vi "Action Message Loop.vi"(7 "Measurement UI Controls":T1 caption="测量UI控件", 8 "error in (no error)":errorcluster caption="错误输入（无错误）", 10 "Data Notifier":refnum<notifier> caption="数据通知器", 11 "Message Queues":T2 caption="消息队列") -> (0 "error out":errorcluster caption="错误输出")   [LabVIEW 2015, in "Action.lvlib"]
doc: "该消息循环负责处理硬件数据采集的相关消息。"
uses:
  Action.lvlib
  <vilib>/Utility/error.llb/Error Cluster From Error Code.vi
  support/Message Queue/Message Queue.lvlib
  support/Message Queue/Enqueue Message (Single).vi
  <vilib>/ErrorRing/Error Ring.xnode
  Acquisition State.ctl
  Hardware Configuration.ctl
  Measure/Measure Type.ctl
  support/Message Queue/Message Cluster.ctl
  support/Message Queue/All Message Queues.ctl
  controls/UI Data.ctl
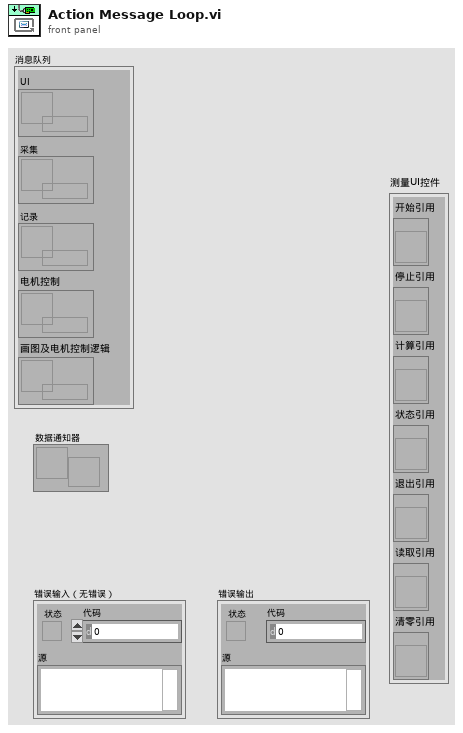
[diagram p1: front panel]
types:
  T1 = typedef "UI Data.ctl" = cluster{"Start Ref":refnum<vi>, "Stop Ref":refnum<vi>, "calculate Ref":refnum<vi>, "Status Ref":refnum<vi>, "Exit Ref":refnum<vi>, "read Ref":refnum<vi>, "clean Ref":refnum<vi>}
  T2 = typedef "Message Queue.lvlib/All Message Queues.ctl" = cluster{"UI":refnum<queue>, "Acquisition":refnum<queue>, "Logging":refnum<queue>, "plot logic":refnum<queue>, "Action Control":refnum<queue>}
  T3 = typedef "Action.lvlib/Hardware Configuration.ctl" = cluster{"PLC设置":T4, "动作设置":T5, "电机设置":T9, "所有测试电机转动逻辑":T10}
  T4 = typedef "Action.lvlib/PLC设置.ctl" = cluster{"ActLogicalStationNumber":i32, "ActUtlType":refnum<k7>}
  T5 = typedef "Action.lvlib/动作设置.ctl" = cluster{"自动跳法测试动作":T6, "其他动作":T8}
  T6 = typedef "Action.lvlib/自动调阀测试动作设置.ctl" = cluster{"夹紧/松阀总":T7, "夹紧/松阀齿":T7, "方向机供油":T7, "扭杆紧/松":T7, "压销":cluster{"PLC指令":T7}}
  T7 = typedef "Action.lvlib/PLC控制指令.ctl" = cluster{"变量类型":u32, "PLC地址":i32, "size":i32, "写入数据(写入时有效)":i16}
  T8 = typedef "Action.lvlib/其他动作设置 .ctl" = cluster{"其他指令1":T7, "其他指令2":T7, "其他指令3":T7, "其他指令4":T7, "其他指令5":T7}
  T9 = typedef "Action.lvlib/电机控制设置.ctl" = cluster{"counter":tag, "方向端口":tag, "当前方向":bool, "频率":dbl, "DAQmx Task":refnum<k21>}
  T10 = typedef "Action.lvlib/所有测试电机转动逻辑.ctl" = cluster{"啮合测试电机转动逻辑":T11, "退回测试电机转动逻辑":T11, "功能测试电机转动逻辑":T11, "力特性测试电机转动逻辑":T11, "自动调阀测试分中电机转动逻辑":T11, "自动调阀测试对中电机转动逻辑":T11}
  T11 = typedef "Action.lvlib/电机转动逻辑1.ctl" = cluster{"反转判断条件1":T12, "停止判断条件1":T13}
  T12 = typedef "Action.lvlib/反转判断条件1.ctl" = cluster{"传感器序号":i32, "条件":enum16{"小于", "大于", "等于"}, "值":dbl, "条件判断时间间隔":i32, "反转等待时长":i32}
  T13 = typedef "Action.lvlib/停止判断条件1.ctl" = cluster{"角度传感器序号":i32, "正转/反转":enum16{"正转", "反转"}, "反转次数":i32, "停止角度":dbl, "停止角度误差范围":dbl}
  T14 = typedef "Measure Type.ctl" = enum16{"啮合", "退回", "功能", "力特性", "内泄漏", "自动调阀测试"}
  T15 = typedef "Action.lvlib/Acquisition State.ctl" = enum16{"Idle", "Acquiring"}
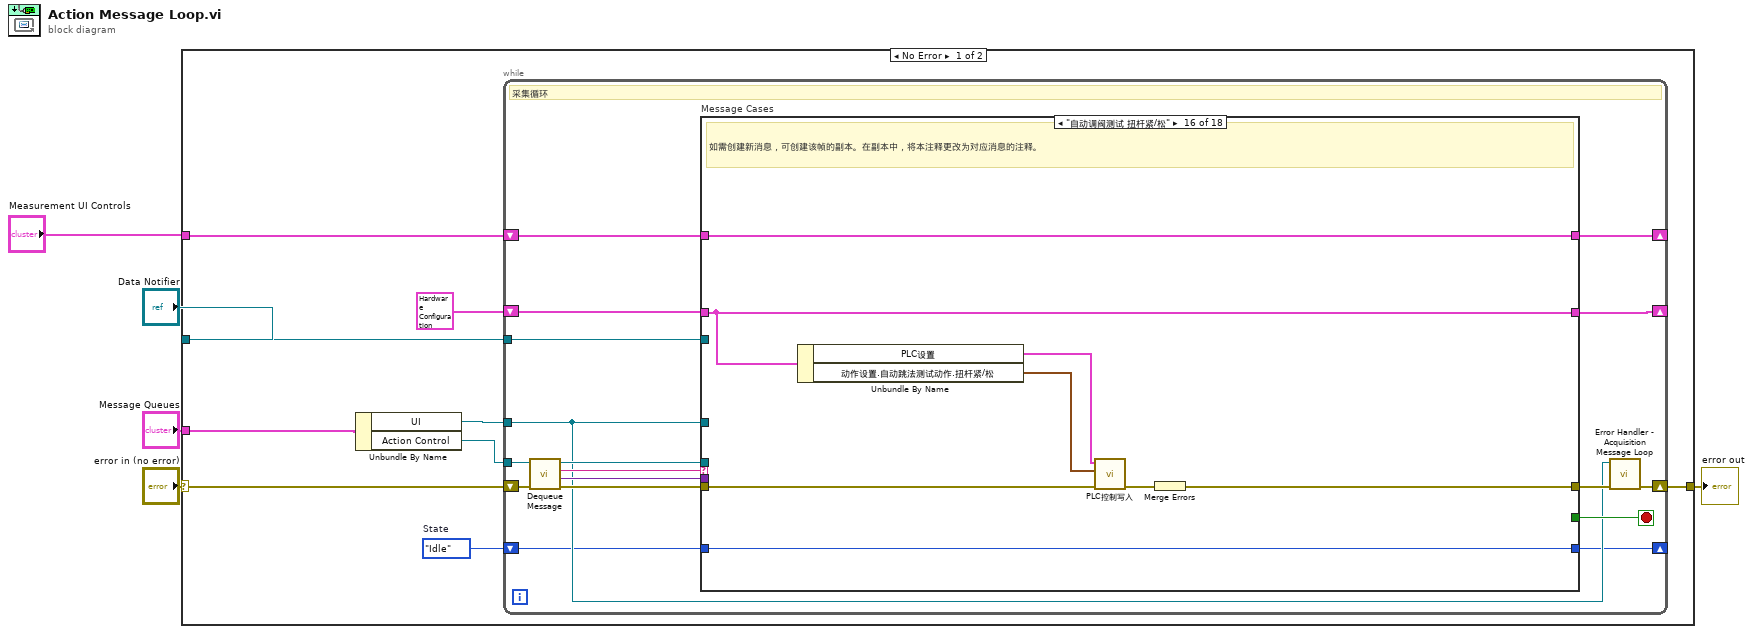
[diagram p0: block diagram]
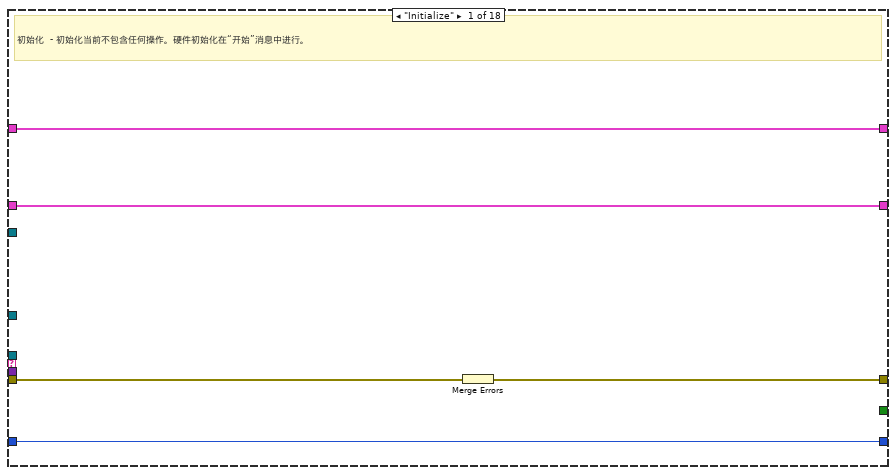
[diagram p2: hidden frame]
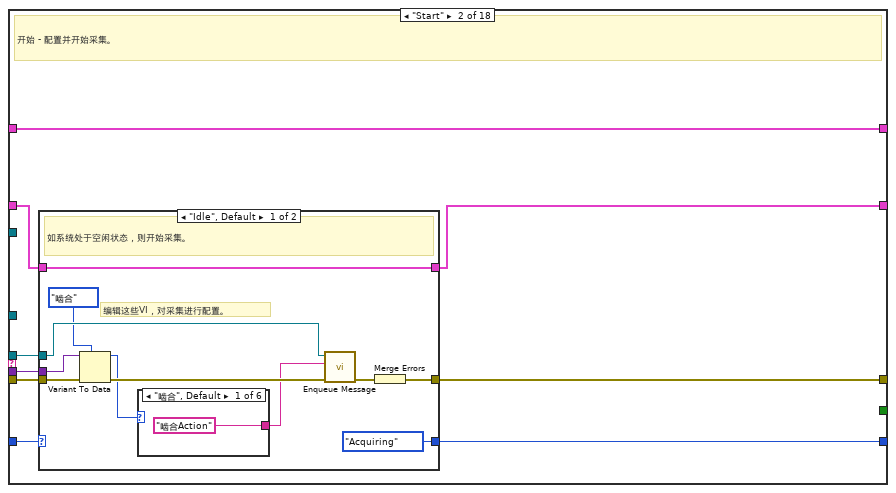
[diagram p3: hidden frame]
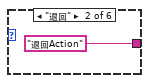
[diagram p4: hidden frame]
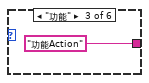
[diagram p5: hidden frame]
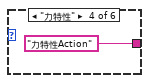
[diagram p6: hidden frame]
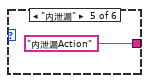
[diagram p7: hidden frame]
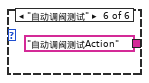
[diagram p8: hidden frame]
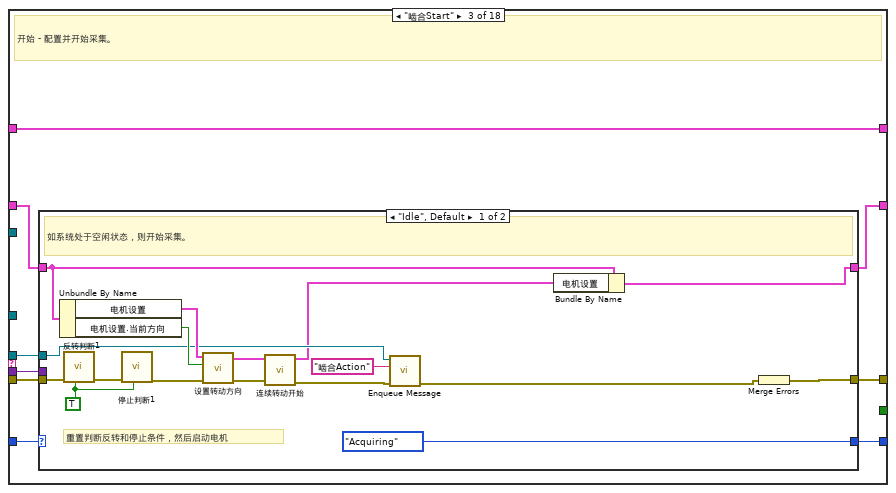
[diagram p10: hidden frame]
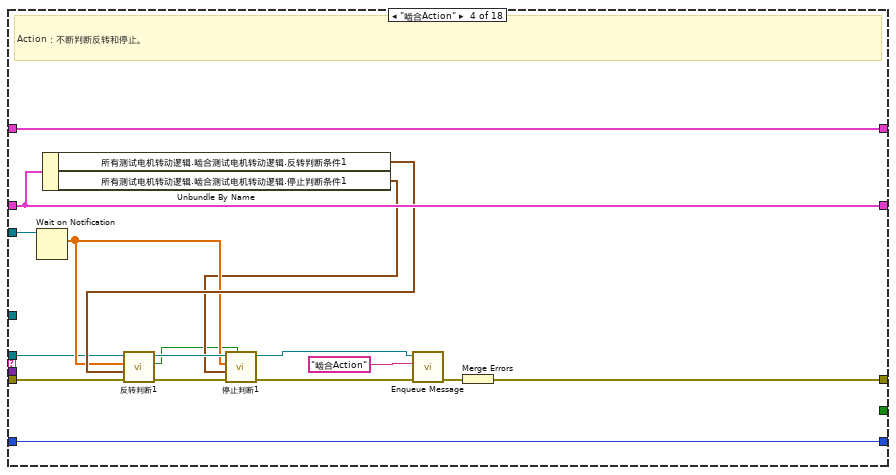
[diagram p12: hidden frame]
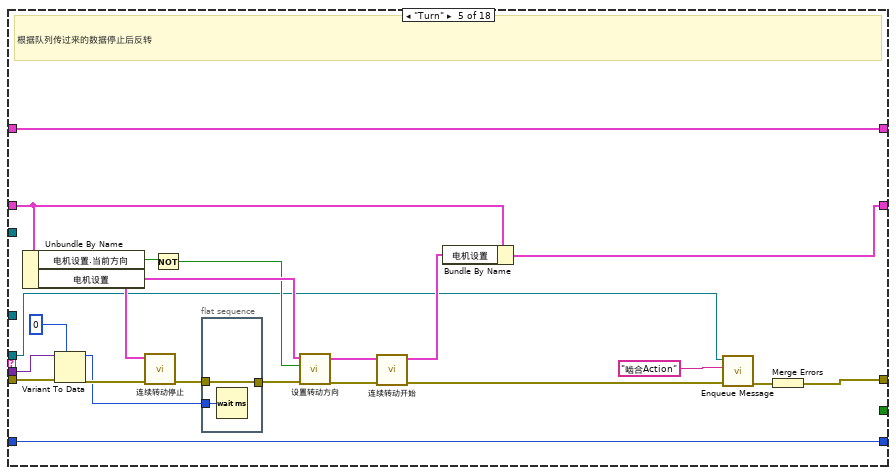
[diagram p13: hidden frame]
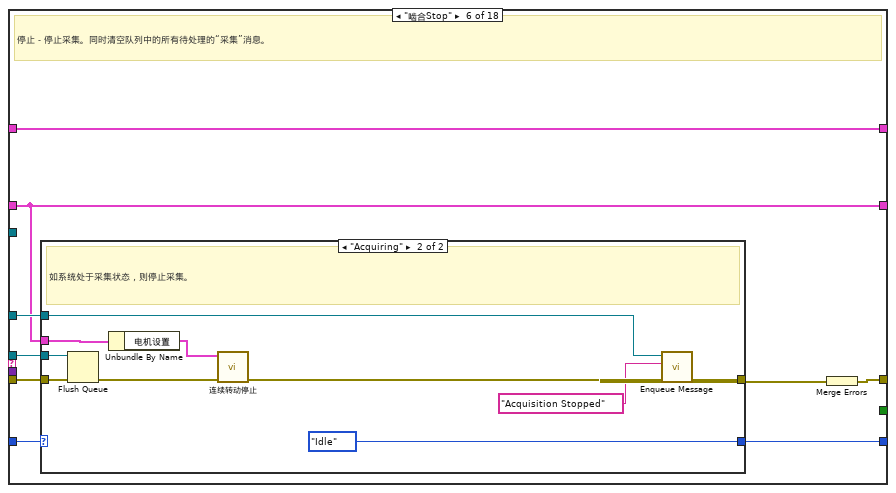
[diagram p14: hidden frame]
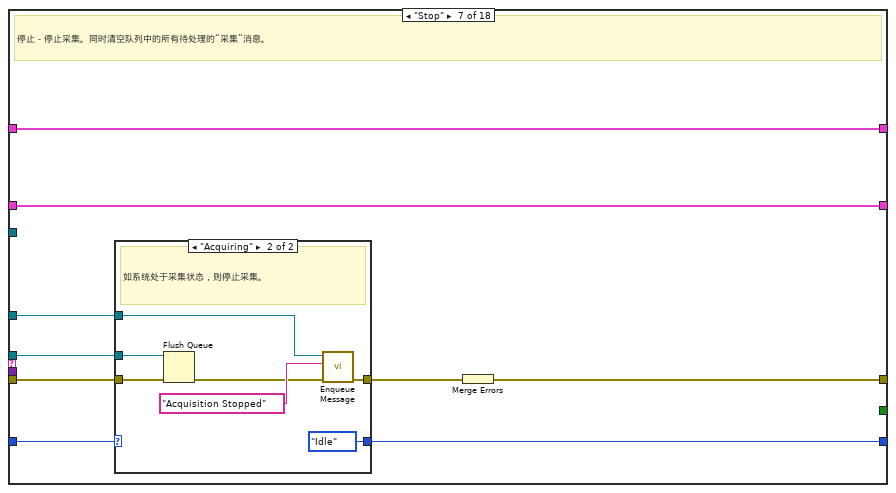
[diagram p16: hidden frame]
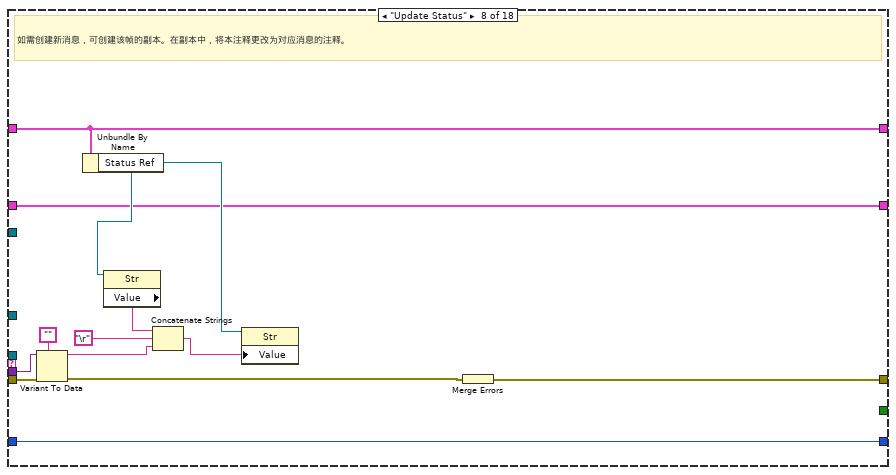
[diagram p18: hidden frame]
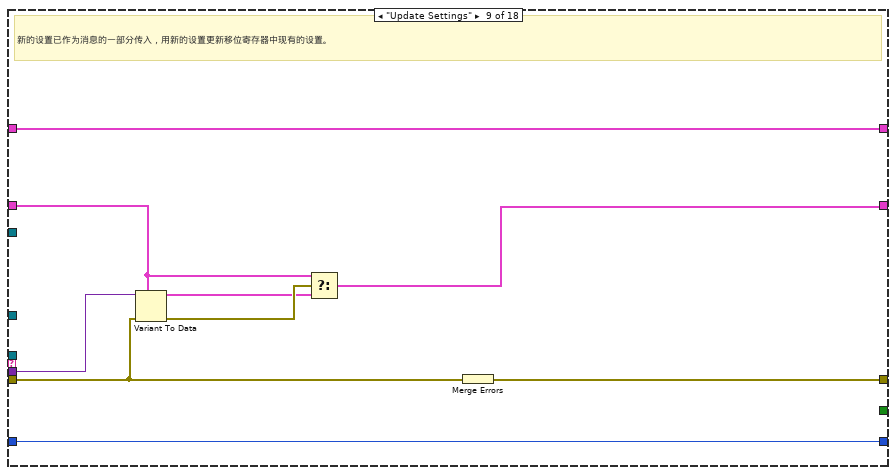
[diagram p19: hidden frame]
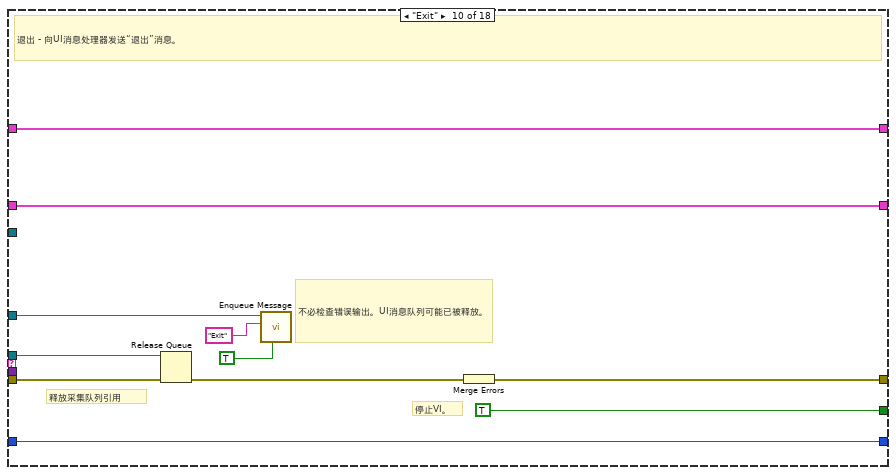
[diagram p20: hidden frame]
diagram:
  n1 = case shown="No Error" "error in (no error)" {
    selector: "error in (no error)" -> [w11 w294]
    tunnel: "Message Queues" -> [w14 _]
    tunnel: [w12 w294] -> w4
    tunnel: "Data Notifier" -> [w9 _]
    tunnel: "Measurement UI Controls" -> [w7 _]
    frame No Error {
      w8 = Acquisition_State."Idle"  # State
      n2 = Unbundle By Name(w14) -> ("UI"=w10:refnum<queue>, "Action Control"=w13:refnum<queue>)
      n3 = while {
        tunnel: w13 -> [w25]
        shift-right: [w22] -> w12
        shift-left: w11 -> [w30]
        tunnel: w10 -> [w21]
        tunnel: w9 -> [w24]
        shift-right: [w19] -> _
        shift-left: w8 -> [w20]
        shift-right: [w15] -> _
        shift-left: w7 -> [w18]
        shift-right: [w16] -> _
        shift-left: T3 {"PLC设置"={"ActLogicalStationNumber"=9600, "ActUtlType"=refnum}, "动作设置"={"自动跳法测试动作"={"夹紧/松阀总"={"变量类型"=2, "PLC地址"=0, "size"=0, "写入数据(写入时有效)"=0}, "夹紧/松阀齿"={"变量类型"=2, "PLC地址"=0, "size"=0, "写入数据(写入时有效)"=0}, "方向机供油"={"变量类型"=2, "PLC地址"=0, "size"=0, "写入数据(写入时有效)"=0}, "扭杆紧/松"={"变量类型"=2, "PLC地址"=0, "size"=0, "写入数据(写入时有效)"=0}, "压销"={"PLC指令"={"变量类型"=2, "PLC地址"=0, "size"=0, "写入数据(写入时有效)"=0}}}, "其他动作"={"其他指令1"={"变量类型"=2, "PLC地址"=0, "size"=0, "写入数据(写入时有效)"=0}, "其他指令2"={"变量类型"=2, "PLC地址"=0, "size"=0, "写入数据(写入时有效)"=0}, "其他指令3"={"变量类型"=2, "PLC地址"=0, "size"=0, "写入数据(写入时有效)"=0}, "其他指令4"={"变量类型"=2, "PLC地址"=0, "size"=0, "写入数据(写入时有效)"=0}, "其他指令5"={"变量类型"=2, "PLC地址"=0, "size"=0, "写入数据(写入时有效)"=0}}}, "电机设置"={"counter"="Dev1/ctr0", "方向端口"="", "当前方向"=FALSE, "频率"=0.0, "DAQmx Task"=""}, "所有测试电机转动逻辑"={"啮合测试电机转动逻辑"={"反转判断条件1"={"传感器序号"=0, "条件"=enum."小于", "值"=0.0, "条件判断时间间隔"=0, "反转等待时长"=0}, "停止判断条件1"={"角度传感器序号"=0, "正转/反转"=enum."正转", "反转次数"=0, "停止角度"=0.0, "停止角度误差范围"=0.0}}, "退回测试电机转动逻辑"={"反转判断条件1"={"传感器序号"=0, "条件"=enum."小于", "值"=0.0, "条件判断时间间隔"=0, "反转等待时长"=0}, "停止判断条件1"={"角度传感器序号"=0, "正转/反转"=enum."正转", "反转次数"=0, "停止角度"=0.0, "停止角度误差范围"=0.0}}, "功能测试电机转动逻辑"={"反转判断条件1"={"传感器序号"=0, "条件"=enum."小于", "值"=0.0, "条件判断时间间隔"=0, "反转等待时长"=0}, "停止判断条件1"={"角度传感器序号"=0, "正转/反转"=enum."正转", "反转次数"=0, "停止角度"=0.0, "停止角度误差范围"=0.0}}, "力特性测试电机转动逻辑"={"反转判断条件1"={"传感器序号"=0, "条件"=enum."小于", "值"=0.0, "条件判断时间间隔"=0, "反转等待时长"=0}, "停止判断条件1"={"角度传感器序号"=0, "正转/反转"=enum."正转", "反转次数"=0, "停止角度"=0.0, "停止角度误差范围"=0.0}}, "自动调阀测试分中电机转动逻辑"={"反转判断条件1"={"传感器序号"=0, "条件"=enum."小于", "值"=0.0, "条件判断时间间隔"=0, "反转等待时长"=0}, "停止判断条件1"={"角度传感器序号"=0, "正转/反转"=enum."正转", "反转次数"=0, "停止角度"=0.0, "停止角度误差范围"=0.0}}, "自动调阀测试对中电机转动逻辑"={"反转判断条件1"={"传感器序号"=0, "条件"=enum."小于", "值"=0.0, "条件判断时间间隔"=0, "反转等待时长"=0}, "停止判断条件1"={"角度传感器序号"=0, "正转/反转"=enum."正转", "反转次数"=0, "停止角度"=0.0, "停止角度误差范围"=0.0}}}} ("Hardware Configuration") -> [w17]
        stop <- w31 stop-if-true
        # "采集循环"
        n4 = call "Dequeue Message.vi"("error in (no error)"=w30, "Message Queue"=w25) -> ("error out"=w29:errorcluster, "Message Data"=w27:variant, "Message"=w28:string, "dup Message Queue"=w26:refnum<queue>)  [unwired: 6 in]
        n5 = case "Message Cases" shown="\"自动调阀测试 扭杆紧/松\"" w28 {
          selector: w28 -> [_ _ _ _ _ _ _ _ _ _ w212 _ _ _ _ _ _ _]
          tunnel: w26 -> [_ w42 w71 w97 w112 w142 w163 _ _ w200 _ _ _ _ _ _ w262 _]
          tunnel: w29 -> [w35 w43 w72 w103 w128 w143 w164 w184 w194 w204 _ w224 w230 w238 w246 w254 w263 w291]
          tunnel: [w36 w45 w74 w111 w133 w144 w165 w187 w196 w206 w211 w223 w232 w240 w248 w256 w265 w293] -> w23
          tunnel: w17 -> [w33 w44 w73 w106 w115 w136 w158 w176 w190 w198 w209 w221 w226 w234 w242 w250 w264 w287]
          tunnel: [_ _ _ _ _ _ _ _ _ TRUE _ _ _ _ _ _ _ _] -> w31
          tunnel: w27 -> [_ w37 w66 _ w127 _ _ w183 w192 _ _ _ _ _ _ _ w257 _]
          tunnel: w21 -> [_ _ _ _ _ w141 w162 _ _ w205 _ _ _ _ _ _ _ _]
          tunnel: w24 -> [_ _ _ w104 _ _ _ _ _ _ _ _ _ _ _ _ _ _]
          tunnel: w20 -> [w34 w41 w70 w108 w130 w140 w161 w186 w193 w199 w210 w222 w231 w239 w247 w255 w261 w292]
          tunnel: [w34 w40 w69 w108 w130 w139 w160 w186 w193 w199 w210 w222 w231 w239 w247 w255 w260 w292] -> w19
          tunnel: w18 -> [w32 w38 w67 w107 w129 w137 w157 w175 w188 w197 w208 w220 w225 w233 w241 w249 w258 w286]
          tunnel: [w33 w39 w68 w106 w113 w136 w158 w176 w189 w198 w209 w221 w226 w234 w242 w250 w259 w287] -> w16
          tunnel: [w32 w38 w67 w107 w129 w137 w157 w175 w188 w197 w208 w220 w225 w233 w241 w249 w258 w286] -> w15
          frame "Initialize" {
            # "初始化  - 初始化当前不包含任何操作。硬件初始化在“开始”消息中进行。"
            n6 = Merge Errors(w35) -> (w36:errorcluster)
          }
          frame "Start" {
            # "开始 - 配置并开始采集。"
            n7 = case shown="\"Idle\", Default" w41 {
              selector: w41 -> [_ w63]
              tunnel: [w56 w65] -> w45
              tunnel: w44 -> [w52 w64]
              tunnel: w43 -> [w51 w65]
              tunnel: w42 -> [w54 _]
              tunnel: [w52 w64] -> w39
              tunnel: [Acquisition_State."Acquiring" ("State") w63] -> w40
              tunnel: w37 -> [w49 _]
              frame "Idle", Default {
                # "编辑这些VI，对采集进行配置。"
                # "如系统处于空闲状态，则开始采集。"
                n8 = Variant To Data(error in=w51, type=Measure_Type."啮合" ("测试类型"), Variant=w49) -> (data=w47:T14, error out=w50:errorcluster)
                n9 = case shown="\"啮合\", Default" w47 {
                  tunnel: ["啮合Action" ("Message") "退回Action" ("Message") "功能Action" ("Message") "力特性Action" ("Message") "内泄漏Action" ("Message") "自动调阀测试Action" ("Message")] -> w46
                  frame "啮合", Default {
                  }
                  frame "退回" {
                  }
                  frame "功能" {
                  }
                  frame "力特性" {
                  }
                  frame "内泄漏" {
                  }
                  frame "自动调阀测试" {
                  }
                }
                n10 = call-poly "Enqueue Message.vi"("error in (no error)"=w50, "Message"=w46, "Message Queue"=w54) -> ("error out"=w55:errorcluster)  [unwired: 7 in, 1 out]
                n11 = Merge Errors(w55) -> (w56:errorcluster)
              }
              frame "Acquiring" {
                # "系统已开始采集。忽略“开始”消息。"
              }
            }
          }
          frame "啮合Start" {
            # "开始 - 配置并开始采集。"
            n12 = case shown="\"Idle\", Default" w70 {
              selector: w70 -> [_ w92]
              tunnel: [w91 w94] -> w74
              tunnel: w73 -> [w77 w93]
              tunnel: w72 -> [w86 w94]
              tunnel: w71 -> [w79 _]
              tunnel: [w75 w93] -> w68
              tunnel: [Acquisition_State."Acquiring" ("State") w92] -> w69
              tunnel: w66 -> [_ _]
              frame "Idle", Default {
                w87 = TRUE ("重置？")
                # "重置判断反转和停止条件，然后启动电机"
                # "如系统处于空闲状态，则开始采集。"
                n13 = Unbundle By Name(w77) -> ("电机设置"=w83:T9, "电机设置.当前方向"=w84:bool)
                n14 = call "反转判断1.vi"("重置？"=w87, "error in (no error)"=w86) -> ("error out"=w88:errorcluster)  [unwired: 7 in, 2 out]
                n15 = call "停止判断1.vi"("重置？"=w87, "error in (no error)"=w88) -> ("error out"=w85:errorcluster)  [unwired: 8 in, 1 out]
                n16 = call "设置转动方向.vi"("error in (no error)"=w85, "方向"=w84, "Hardware Resources in"=w83) -> ("error out"=w82:errorcluster, "Hardware Resources out"=w81:T9)  [unwired: 7 in]
                n17 = call "连续转动开始.vi"("error in (no error)"=w82, "Hardware Resources in"=w81) -> ("error out"=w80:errorcluster, "Hardware Resources out"=w76:T9)  [unwired: 8 in]
                n18 = call-poly "Enqueue Message.vi"("error in (no error)"=w80, "Message"="啮合Action", "Message Queue"=w79) -> ("error out"=w78:errorcluster)  [unwired: 7 in, 1 out]
                n19 = Bundle By Name(cluster=w77, "电机设置"=w76) -> (w75:T3)
                n20 = Merge Errors(w78) -> (w91:errorcluster)
              }
              frame "Acquiring" {
                # "系统已开始采集。忽略“开始”消息。"
              }
            }
          }
          frame "啮合Action" {
            # "Action：不断判断反转和停止。"
            n21 = Wait on Notification(notifier=w104) -> (notification=w100:dbl[])  [unwired: 3 in, 3 out]
            n22 = Unbundle By Name(w106) -> ("所有测试电机转动逻辑.啮合测试电机转动逻辑.反转判断条件1"=w105:T12, "所有测试电机转动逻辑.啮合测试电机转动逻辑.停止判断条件1"=w99:T13)
            n23 = call "反转判断1.vi"("error in (no error)"=w103, "反转判断条件1"=w105, "传感器数据"=w100, "Message Queue"=w97) -> ("error out"=w102:errorcluster, "反转"=w98:bool, "Message Queue 2"=w101:refnum<queue>)  [unwired: 5 in]
            n24 = call "停止判断1.vi"("反转？"=w98, "error in (no error)"=w102, "反转判断条件1"=w99, "传感器数据"=w100, "Message Queue"=w101) -> ("error out"=w95:errorcluster, "Message Queue 2"=w96:refnum<queue>)  [unwired: 5 in]
            n25 = call-poly "Enqueue Message.vi"("error in (no error)"=w95, "Message"="啮合Action", "Message Queue"=w96) -> ("error out"=w110:errorcluster)  [unwired: 7 in, 1 out]
            n26 = Merge Errors(w110) -> (w111:errorcluster)
          }
          frame "Turn" {
            # "根据队列传过来的数据停止后反转"
            n27 = Unbundle By Name(w115) -> ("电机设置.当前方向"=w120:bool, "电机设置"=w121:T9)
            n28 = Variant To Data(error in=w128, type=0, Variant=w127) -> (data=w124:i32, error out=w125:errorcluster)
            n29 = call "连续转动停止.vi"("error in (no error)"=w125, "Hardware Resources in"=w121) -> ("error out"=w123:errorcluster)  [unwired: 9 in]
            n30 = Not(x=w120) -> (.not. x?=w119:bool)
            n31 = flat-sequence {
              tunnel: w124 -> [w135]
              tunnel: [w134] -> w122
              tunnel: w123 -> [w134]
              frame #0 {
                n32 = Wait (ms)(milliseconds to wait=w135) -> ()  [unwired: 1 out]
              }
            }
            n33 = call "设置转动方向.vi"("error in (no error)"=w122, "方向"=w119, "Hardware Resources in"=w121) -> ("error out"=w118:errorcluster, "Hardware Resources out"=w117:T9)  [unwired: 7 in]
            n34 = call "连续转动开始.vi"("error in (no error)"=w118, "Hardware Resources in"=w117) -> ("error out"=w116:errorcluster, "Hardware Resources out"=w114:T9)  [unwired: 8 in]
            n35 = Bundle By Name(cluster=w115, "电机设置"=w114) -> (w113:T3)
            n36 = call-poly "Enqueue Message.vi"("error in (no error)"=w116, "Message"="啮合Action", "Message Queue"=w112) -> ("error out"=w132:errorcluster)  [unwired: 7 in, 1 out]
            n37 = Merge Errors(w132) -> (w133:errorcluster)
          }
          frame "啮合Stop" {
            # "停止－停止采集。同时清空队列中的所有待处理的“采集”消息。"
            n38 = case shown="\"Acquiring\"" w140 {
              selector: w140 -> [w146 _]
              tunnel: w143 -> [w145 w156]
              tunnel: w142 -> [_ w155]
              tunnel: w141 -> [_ w154]
              tunnel: [w146 Acquisition_State."Idle" ("State")] -> w139
              tunnel: [w145 w153] -> w138
              tunnel: w136 -> [_ w149]
              frame "Idle", Default {
                # "系统已处于空闲状态。忽略“停止”消息。"
              }
              frame "Acquiring" {
                # "如系统处于采集状态，则停止采集。"
                n39 = Flush Queue(queue=w155, error in (no error)=w156) -> (error out=w150:errorcluster)  [unwired: 2 out]
                n40 = Unbundle By Name(w149) -> ("电机设置"=w148:T9)
                n41 = call "连续转动停止.vi"("error in (no error)"=w150, "Hardware Resources in"=w148) -> ("error out"=w147:errorcluster)  [unwired: 9 in]
                n42 = call-poly "Enqueue Message.vi"("error in (no error)"=w147, "Message"="Acquisition Stopped", "Message Queue"=w154) -> ("error out"=w153:errorcluster)  [unwired: 7 in, 1 out]
              }
            }
            n43 = Merge Errors(w138) -> (w144:errorcluster)
          }
          frame "Stop" {
            # "停止－停止采集。同时清空队列中的所有待处理的“采集”消息。"
            n44 = case shown="\"Acquiring\"" w161 {
              selector: w161 -> [w167 _]
              tunnel: w164 -> [w166 w174]
              tunnel: w163 -> [_ w173]
              tunnel: w162 -> [_ w172]
              tunnel: [w167 Acquisition_State."Idle" ("State")] -> w160
              tunnel: [w166 w171] -> w159
              frame "Idle", Default {
                # "系统已处于空闲状态。忽略“停止”消息。"
              }
              frame "Acquiring" {
                # "如系统处于采集状态，则停止采集。"
                n45 = Flush Queue(queue=w173, error in (no error)=w174) -> (error out=w168:errorcluster)  [unwired: 2 out]
                n46 = call-poly "Enqueue Message.vi"("error in (no error)"=w168, "Message"="Acquisition Stopped", "Message Queue"=w172) -> ("error out"=w171:errorcluster)  [unwired: 7 in, 1 out]
              }
            }
            n47 = Merge Errors(w159) -> (w165:errorcluster)
          }
          frame "Update Status" {
            # "如需创建新消息，可创建该帧的副本。在副本中，将本注释更改为对应消息的注释。"
            n48 = Variant To Data(error in=w184, type="", Variant=w183) -> (data=w178:string, error out=w182:errorcluster)
            n49 = Unbundle By Name(w175) -> ("Status Ref"=w181:refnum<vi>)
            n50 = property class="Str"(reference=w181) -> ("Value"=w180:string)  [unwired: 1 in, 2 out]
            n51 = Concatenate Strings(w180, "\r", w178) -> (w177:string)
            n52 = property class="Str"(reference=w181, "Value"=w177) -> ()  [unwired: 1 in, 2 out]
            n53 = Merge Errors(w182) -> (w187:errorcluster)
          }
          frame "Update Settings" {
            # "新的设置已作为消息的一部分传入，用新的设置更新移位寄存器中现有的设置。"
            n54 = Variant To Data(error in=w194, type=w190, Variant=w192) -> (data=w191:T3, error out=w195:errorcluster)
            n55 = Select(t=w190, s=w195, f=w191) -> (s? t:f=w189:T3)
            n56 = Merge Errors(w194) -> (w196:errorcluster)
          }
          frame "Exit" {
            # "不必检查错误输出。UI消息队列可能已被释放。"
            # "释放采集队列引用"
            # "停止VI。"
            # "退出 - 向UI消息处理器发送“退出”消息。"
            n57 = Release Queue(queue=w200, error in (no error)=w204) -> (error out=w201:errorcluster)  [unwired: 1 in, 2 out]
            n58 = call-poly "Enqueue Message.vi"("Priority Message? (F)"=TRUE, "Message"="Exit", "Message Queue"=w205) -> ()  [unwired: 7 in, 2 out]
            n59 = Merge Errors(w201) -> (w206:errorcluster)
          }
          frame Default {
            # "如得到的消息未经任何分支定义，则运行“默认”分支。输出程序错误。"
            n60 = xnode "Error Ring"("parameter 0"=w212) -> ("error out"=w211:errorcluster)
          }
          frame "---Copy This Frame---" {
            # "如需创建新消息，可创建该帧的副本。在副本中，将本注释更改为对应消息的注释。"
            n61 = Merge Errors(w224) -> (w223:errorcluster)
          }
          frame "自动调阀测试 夹紧/松阀总" {
            # "如需创建新消息，可创建该帧的副本。在副本中，将本注释更改为对应消息的注释。"
            n62 = Unbundle By Name(w226) -> ("PLC设置"=w228:T4, "动作设置.自动跳法测试动作.夹紧/松阀总"=w227:T7)
            n63 = call "PLC控制写入.vi"("error in (no error)"=w230, "PLC指令"=w227, "PLC设置"=w228) -> ("error out"=w229:errorcluster)  [unwired: 6 in, 2 out]
            n64 = Merge Errors(w229) -> (w232:errorcluster)
          }
          frame "自动调阀测试 夹紧/松阀齿" {
            # "如需创建新消息，可创建该帧的副本。在副本中，将本注释更改为对应消息的注释。"
            n65 = Unbundle By Name(w234) -> ("PLC设置"=w236:T4, "动作设置.自动跳法测试动作.夹紧/松阀齿"=w235:T7)
            n66 = call "PLC控制写入.vi"("error in (no error)"=w238, "PLC指令"=w235, "PLC设置"=w236) -> ("error out"=w237:errorcluster)  [unwired: 6 in, 2 out]
            n67 = Merge Errors(w237) -> (w240:errorcluster)
          }
          frame "自动调阀测试 方向机供油" {
            # "如需创建新消息，可创建该帧的副本。在副本中，将本注释更改为对应消息的注释。"
            n68 = Unbundle By Name(w242) -> ("PLC设置"=w244:T4, "动作设置.自动跳法测试动作.方向机供油"=w243:T7)
            n69 = call "PLC控制写入.vi"("error in (no error)"=w246, "PLC指令"=w243, "PLC设置"=w244) -> ("error out"=w245:errorcluster)  [unwired: 6 in, 2 out]
            n70 = Merge Errors(w245) -> (w248:errorcluster)
          }
          frame "自动调阀测试 扭杆紧/松" {
            # "如需创建新消息，可创建该帧的副本。在副本中，将本注释更改为对应消息的注释。"
            n71 = Unbundle By Name(w250) -> ("PLC设置"=w252:T4, "动作设置.自动跳法测试动作.扭杆紧/松"=w251:T7)
            n72 = call "PLC控制写入.vi"("error in (no error)"=w254, "PLC指令"=w251, "PLC设置"=w252) -> ("error out"=w253:errorcluster)  [unwired: 6 in, 2 out]
            n73 = Merge Errors(w253) -> (w256:errorcluster)
          }
          frame "自动调阀测试_分中Start" {
            # "开始 - 配置并开始采集。"
            n74 = case shown="\"Idle\", Default" w261 {
              selector: w261 -> [_ w283]
              tunnel: [w282 w285] -> w265
              tunnel: w264 -> [w268 w284]
              tunnel: w263 -> [w277 w285]
              tunnel: w262 -> [w270 _]
              tunnel: [w266 w284] -> w259
              tunnel: [Acquisition_State."Acquiring" ("State") w283] -> w260
              tunnel: w257 -> [_ _]
              frame "Idle", Default {
                w278 = TRUE ("重置？")
                # "重置判断反转和停止条件，然后启动电机"
                # "如系统处于空闲状态，则开始采集。"
                n75 = Unbundle By Name(w268) -> ("电机设置"=w274:T9, "电机设置.当前方向"=w275:bool)
                n76 = call "反转判断1.vi"("重置？"=w278, "error in (no error)"=w277) -> ("error out"=w279:errorcluster)  [unwired: 7 in, 2 out]
                n77 = call "停止判断1.vi"("重置？"=w278, "error in (no error)"=w279) -> ("error out"=w276:errorcluster)  [unwired: 8 in, 1 out]
                n78 = call "设置转动方向.vi"("error in (no error)"=w276, "方向"=w275, "Hardware Resources in"=w274) -> ("error out"=w273:errorcluster, "Hardware Resources out"=w272:T9)  [unwired: 7 in]
                n79 = call "连续转动开始.vi"("error in (no error)"=w273, "Hardware Resources in"=w272) -> ("error out"=w271:errorcluster, "Hardware Resources out"=w267:T9)  [unwired: 8 in]
                n80 = call-poly "Enqueue Message.vi"("error in (no error)"=w271, "Message"="啮合Action", "Message Queue"=w270) -> ("error out"=w269:errorcluster)  [unwired: 7 in, 1 out]
                n81 = Bundle By Name(cluster=w268, "电机设置"=w267) -> (w266:T3)
                n82 = Merge Errors(w269) -> (w282:errorcluster)
              }
              frame "Acquiring" {
                # "系统已开始采集。忽略“开始”消息。"
              }
            }
          }
          frame "自动调阀测试_分中monitor" {
            # "如需创建新消息，可创建该帧的副本。在副本中，将本注释更改为对应消息的注释。"
            n83 = Unbundle By Name(w287) -> ("PLC设置"=w289:T4, "PLC指令"=w288:T7)
            n84 = call "PLC控制写入.vi"("error in (no error)"=w291, "PLC指令"=w288, "PLC设置"=w289) -> ("error out"=w290:errorcluster)  [unwired: 6 in, 2 out]
            n85 = Merge Errors(w290) -> (w293:errorcluster)
          }
        }
        n86 = call "Error Handler - Acquisition Message Loop.vi"("error in (no error)"=w23, "Message Queue"=w21) -> ("dup error in"=w22:errorcluster)  [unwired: 8 in, 1 out]
      }
    }
    frame Error {
    }
  }
  "error out" <- w4
